vi "Get Requested Ground Intake Controls.vi"(0 "Driver Axes":dbl[](array[numeric]), 5 "Driver Buttons":bool[](array[boolean]), 9 "Deadband":dbl=0.2 format="%#_13g") -> (3 "Intake Command Requested?":bool, 4 "Intake Sideways Cone Requested?":bool, 6 "Intake Cube Requested?":bool, 10 "Outtake Requested?":bool, 12 "Intake Cone Feeder":bool, 14 "Intake Cube Feeder":bool, 15 "Intake Upright Cone Requested?":bool)   [LabVIEW 2020]
uses:
  <vilib>/Rock Robotics/WPI/Joystick/XBox Buttons Indexer.ctl
  <vilib>/Rock Robotics/WPI/Joystick/XBox Axes Indexer.ctl
  <vilib>/Rock Robotics/WPI/Utilities/WPI_GetSetVariantRefNum.vi
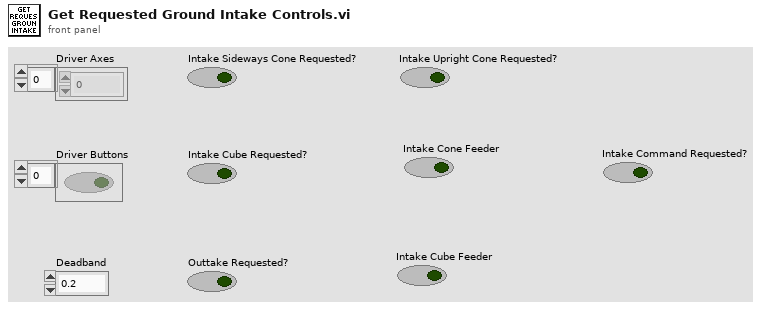
[diagram p1: front panel]
types:
  T1 = typedef "XBox Buttons Indexer.ctl" = enum16{"A", "B", "X", "Y", "Left Bumper", "Right Bumper", "Back", "Start", "Left Joystick", "Right Joystick"}
  T2 = typedef "XBox Axes Indexer.ctl" = enum16{"Left X", "Left Y", "Left Trigger", "Right Trigger", "Right X", "Right Y"}
  T3 = typedef "WPI_JoystickDevRef.ctl" = cluster{"Device":T4}
  T4 = typedef "WPI_JoystickDeviceEnum.ctl" = enum16{"USB 0", "USB 1", "USB 2", "USB 3", "USB 4", "USB 5"}
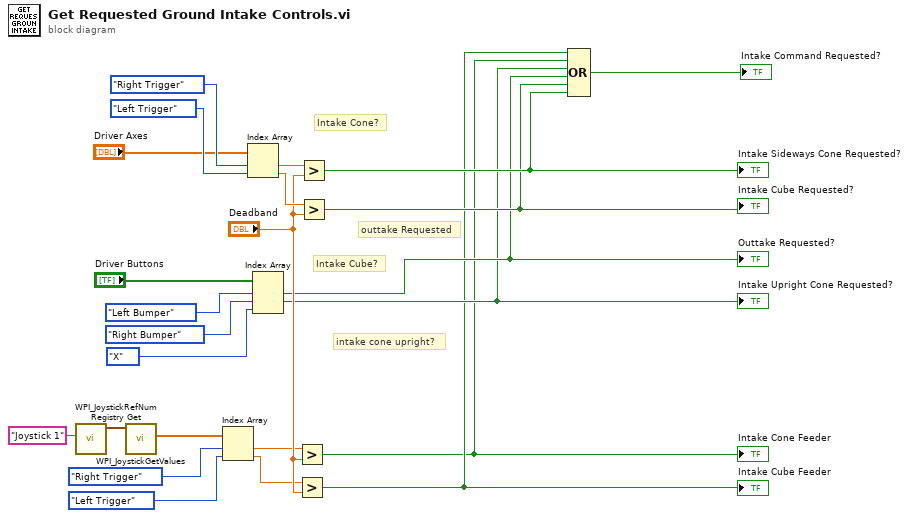
[diagram p0: block diagram]
diagram:
  # "outtake Requested"
  # "intake cone upright?"
  # "Intake Cube?"
  # "Intake Cone?"
  n1 = call <vilib>:"WPI_JoystickRefNum Registry Get.vi"("refnum name"="Joystick 1") -> ("JoystickDevRef"=w17:T3)  [unwired: 1 in, 9 out]
  n2 = call <vilib>:"WPI_JoystickGetValues.vi"("JoystickDevRef"=w17) -> ("Axes"=w15:dbl[])  [unwired: 6 in, 4 out]
  n3 = Index Array(array=w15, index #1=XBox_Axes_Indexer."Right Trigger" ("XBox Axes"), index #2=XBox_Axes_Indexer."Left Trigger" ("XBox Axes")) -> (element #1=w10:dbl, element #2=w11:dbl)
  n4 = Index Array(array="Driver Axes", index #1=XBox_Axes_Indexer."Right Trigger" ("XBox Axes"), index #2=XBox_Axes_Indexer."Left Trigger" ("XBox Axes")) -> (element #1=w21:dbl, element #2=w20:dbl)
  n5 = Index Array(array="Driver Buttons", index #1=XBox_Buttons_Indexer."Left Bumper" ("XBox Buttons"), index #2=XBox_Buttons_Indexer."Right Bumper" ("XBox Buttons"), index #3=XBox_Buttons_Indexer."X" ("XBox Buttons")) -> (element #1=w6:bool, element #2=w5:bool)  [unwired: 1 out]
  "Outtake Requested?" <- w6
  "Intake Upright Cone Requested?" <- w5
  n6 = Greater?(x=w10, y="Deadband") -> (0:w1:bool)
  "Intake Cone Feeder" <- w1
  n7 = Greater?(x=w11, y="Deadband") -> (0:w4:bool)
  "Intake Cube Feeder" <- w4
  n8 = Greater?(x=w21, y="Deadband") -> (0:w8:bool)
  "Intake Sideways Cone Requested?" <- w8
  n9 = Greater?(x=w20, y="Deadband") -> (0:w7:bool)
  "Intake Cube Requested?" <- w7
  n10 = Compound Arithmetic op=OR(w4, w1, w5, w6, w7, w8) -> (→"Intake Command Requested?":bool)
